vi "Configure Frequency (Center Span).vi"(8 "error in (no error)":errorcluster, 9 "Span (2 GHz)":dbl=2000000000.0, 10 "Center Frequency (1 GHz)":dbl=1000000000.0 format="%#.6g", 11 "VISA resource name":refnum<visa-resource-name>) -> (0 "error out":errorcluster, 3 "VISA resource name out":refnum<visa-resource-name>)   [LabVIEW 2013, in "Template - Spectrum Analyzer.lvlib"]
doc: "Configures the frequency range of the spectrum analyzer using the center frequency and the frequency span. If span corresponds to zero Hertz, then the spectrum analyzer operates in time-domain mode. Otherwise, spectrum analyzer operates in frequency-domain mode.\n\n Frequency Start = Center Frequency - Span/2\n Frequency Stop = Center Frequency + Span/2"
uses:
  <instrlib>/_Template - Spectrum Analyzer/Template - Spectrum Analyzer.lvlib
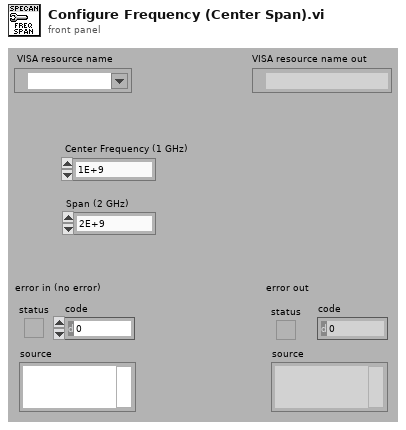
[diagram p1: front panel]
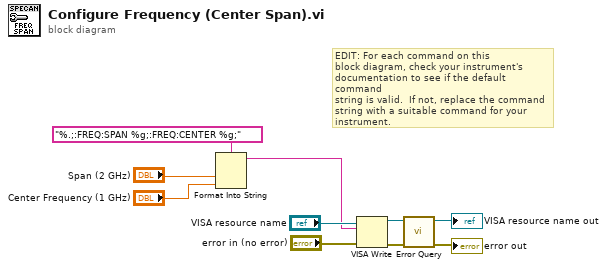
[diagram p0: block diagram]
diagram:
  # "EDIT: For each command on this\nblock diagram, check your instrument's\ndocumentation to see if the default command\nstring is valid.  If not, replace the command\nstring with a suitable command for your\ninstrument."
  n1 = Format Into String(format string="%.;:FREQ:SPAN %g;:FREQ:CENTER %g;", "Span (2 GHz)", "Center Frequency (1 GHz)") -> (resulting string=w8:string)  [unwired: 2 in, 1 out]
  n2 = VISA Write(VISA resource name="VISA resource name", write buffer=w8, error in (no error)="error in (no error)") -> (VISA resource name out=w4:refnum<visa-resource-name>, error out=w2:errorcluster)  [unwired: 1 out]
  n3 = call <instrlib>:"Error Query.vi"("error in (no error)"=w2, "VISA resource name"=w4) -> ("error out"=→"error out":errorcluster, "VISA resource name out"=→"VISA resource name out":refnum<visa-resource-name>)  [unwired: 6 in, 2 out]
